vi "ErrorCheckHWI.vi"(8 "error in (no error)":errorcluster, 11 "SRS_SG380 in":refnum<class "SRS_SG380.lvclass">) -> (0 "error out":errorcluster, 3 "SRS_SG380 out":refnum<class "SRS_SG380.lvclass">)   [LabVIEW 2013, in "SRS_SG380.lvclass"]
uses:
  SRS_SG380.lvclass
  SRS_SG380.lvclass/SRS_SG380.ctl
  <vilib>/Utility/error.llb/DialogType.ctl
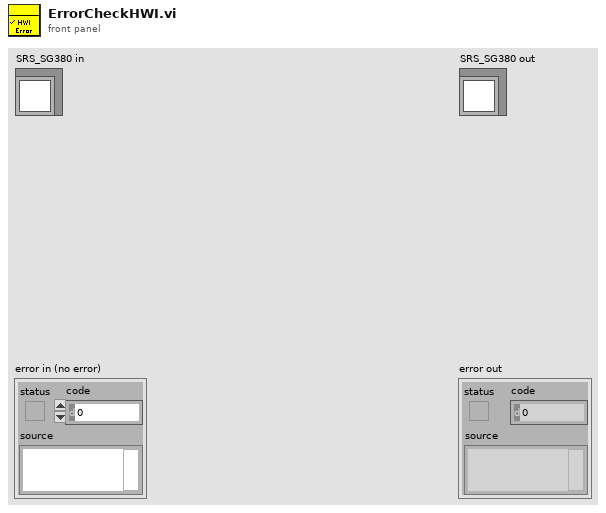
[diagram p1: front panel]
types:
  T1 = typedef "DialogType.ctl" = u16
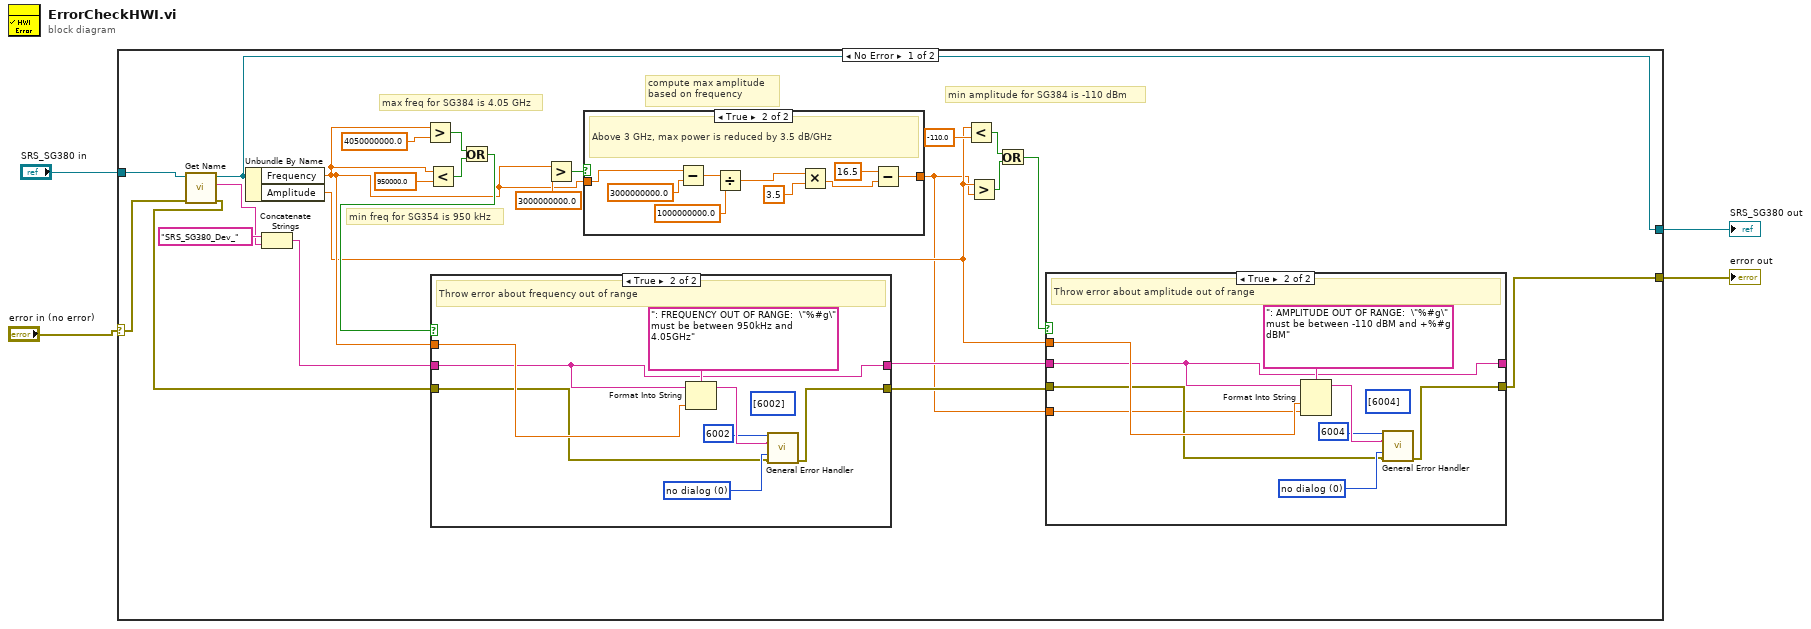
[diagram p0: block diagram]
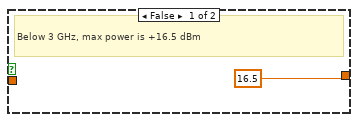
[diagram p2: hidden frame]
diagram:
  n1 = case shown="No Error" "error in (no error)" {
    selector: "error in (no error)" -> [w27 w60]
    tunnel: "SRS_SG380 in" -> [w28 w61]
    tunnel: [w6 w60] -> w2
    tunnel: [w5 w61] -> w1
    frame No Error {
      # "compute max amplitude\nbased on frequency"
      # "min amplitude for SG384 is -110 dBm"
      # "min freq for SG354 is 950 kHz"
      # "max freq for SG384 is 4.05 GHz"
      n2 = call-dynamic "Get Name.vi"("error in (no error)"=w27, "Device in"=w28) -> ("error out"=w18:errorcluster, "Name"=w25:string, "Device out"=w5:refnum<class "SRS_SG380.lvclass">)  [unwired: 7 in]
      n3 = Unbundle By Name(w5) -> ("Frequency"=w14:dbl, "Amplitude"=w10:dbl)
      n4 = Concatenate Strings("SRS_SG380_Dev_" ("string"), w25) -> (w19:string)
      n5 = Greater?(x=w14, y=4050000000.0) -> (0:w21:bool)
      n6 = Less?(x=w14, y=950000.0) -> (x < y?=w22:bool)
      n7 = Or(x=w21, y=w22) -> (x .or. y?=w20:bool)
      n8 = case shown="True" w20 {
        tunnel: w18 -> [w51 w55]
        tunnel: w14 -> [_ w58]
        tunnel: [w51 w53] -> w8
        tunnel: w19 -> [w50 w52]
        tunnel: [w50 w52] -> w9
        frame False {
        }
        frame True {
          (unwired) i32[] [6002] ("[user-defined codes]")
          w56 = T1 0 items=["no dialog", "OK message", "continue or stop message", "OK message + warnings", "continue/stop + warnings"] ("type of dialog (OK msg:1)")
          # "Throw error about frequency out of range"
          n9 = Format Into String(format string=": FREQUENCY OUT OF RANGE:  \"%#g\" must be between 950kHz and 4.05GHz", initial string=w52, w58) -> (resulting string=w57:string)  [unwired: 1 in, 1 out]
          n10 = call <vilib>:"General Error Handler.vi"("[error code] (0)"=6002 ("error code (no error:0)"), "[error source] (\" \")"=w57, "type of dialog (OK msg:1)"=w56, "error in (no error)"=w55) -> ("error out"=w53:errorcluster)  [unwired: 7 in, 4 out]
        }
      }
      n11 = Greater?(x=w14, y=3000000000.0) -> (0:w16:bool)
      n12 = case shown="True" w16 {
        tunnel: w14 -> [_ w38]
        tunnel: [16.5 w33] -> w7
        frame False {
          # "Below 3 GHz, max power is +16.5 dBm"
        }
        frame True {
          # "Above 3 GHz, max power is reduced by 3.5 dB/GHz"
          n13 = Subtract(x=w38, y=3000000000.0) -> (x-y=w32:dbl)
          n14 = Divide(x=w32, y=1000000000.0) -> (x/y=w30:dbl)
          n15 = Multiply(x=w30, y=3.5) -> (x*y=w34:dbl)
          n16 = Subtract(x=16.5, y=w34) -> (x-y=w33:dbl)
        }
      }
      n17 = Less?(x=w10, y=-110.0) -> (x < y?=w12:bool)
      n18 = Greater?(x=w10, y=w7) -> (0:w13:bool)
      n19 = Or(x=w12, y=w13) -> (x .or. y?=w11:bool)
      n20 = case shown="True" w11 {
        tunnel: w8 -> [w40 w45]
        tunnel: w10 -> [_ w48]
        tunnel: [w40 w43] -> w6
        tunnel: w9 -> [w39 w42]
        tunnel: [w39 w42] -> _
        tunnel: w7 -> [_ w41]
        frame False {
        }
        frame True {
          (unwired) i32[] [6004] ("[user-defined codes]")
          w46 = T1 0 items=["no dialog", "OK message", "continue or stop message", "OK message + warnings", "continue/stop + warnings"] ("type of dialog (OK msg:1)")
          # "Throw error about amplitude out of range"
          n21 = Format Into String(format string=": AMPLITUDE OUT OF RANGE:  \"%#g\" must be between -110 dBM and +%#g dBM", initial string=w42, w48, w41) -> (resulting string=w47:string)  [unwired: 1 in, 1 out]
          n22 = call <vilib>:"General Error Handler.vi"("[error code] (0)"=6004 ("error code (no error:0)"), "[error source] (\" \")"=w47, "type of dialog (OK msg:1)"=w46, "error in (no error)"=w45) -> ("error out"=w43:errorcluster)  [unwired: 7 in, 4 out]
        }
      }
    }
    frame Error {
    }
  }
  "error out" <- w2
  "SRS_SG380 out" <- w1
